vi "Recall Waveform to Reference Channel.vi"(7 "Waveform File":string, 8 "error in (no error)":errorcluster, 9 "Reference Channel (0: Reference 1)":i32(ring) items=["Reference 1", "Reference 2", "Reference 3", "Reference 4", "Edit Memory"], 10 "Source Waveform (0: Arbitrary Memory 1)":i32(ring) items=["Arbitrary Memory 1", "Arbitrary Memory 2", "Arbitrary Memory 3", "Arbitrary Memory 4", "Waveform File"], 11 "VISA resource name":refnum<visa-resource-name>) -> (0 "error out":errorcluster, 3 "VISA resource name out":refnum<visa-resource-name>)   [LabVIEW 2017, in "Scope.lvlib" / "Tektronix DPO MSO 2000 4000 Series.lvlib"]
doc: "Recalls a stored waveform to a reference memory location.\n\n<B>Notes:</B>\n(1) Only the first waveform in a .CSV file is recalled for multiple waveform .CSV files. \n\n(2) Recall of digital waveforms (D0 through D15) is not supported.\n\n(3) For MDO3000 series models, a saved ARB waveform cannot be recalled to a reference location. It can only be recalled to an EMEM location. However, an AFG waveform can be recalled into either a reference or EMEM location."
uses:
  Tektronix DPO MSO 2000 4000 Series.lvlib
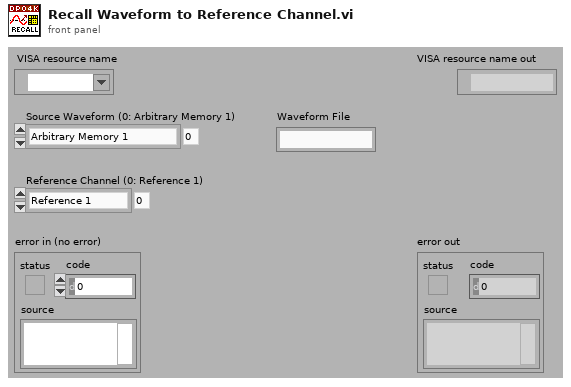
[diagram p1: front panel]
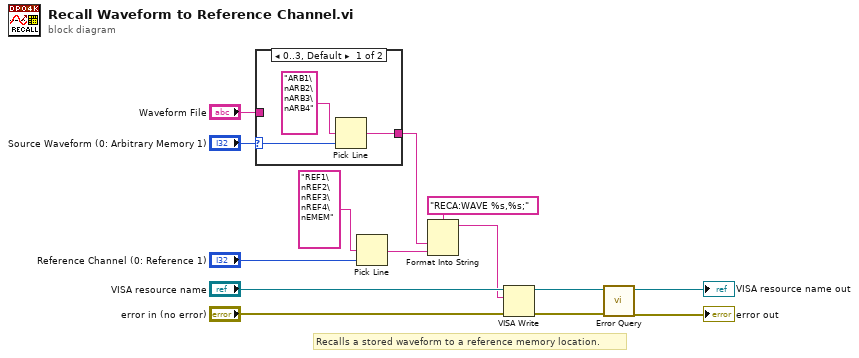
[diagram p0: block diagram]
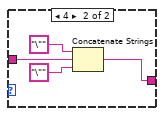
[diagram p2: hidden frame]
diagram:
  # "Recalls a stored waveform to a reference memory location."
  n1 = case shown="0..3, Default" "Source Waveform (0: Arbitrary Memory 1)" {
    selector: "Source Waveform (0: Arbitrary Memory 1)" -> [w16 _]
    tunnel: "Waveform File" -> [_ w21]
    tunnel: [w15 w18] -> w3
    frame 0..3, Default {
      n2 = Pick Line(multi-line string="ARB1\nARB2\nARB3\nARB4", line index=w16) -> (output string=w15:string)  [unwired: 1 in]
    }
    frame 4 {
      n3 = Concatenate Strings("\"" ("string"), w21, "\"" ("string")) -> (w18:string)
    }
  }
  n4 = Pick Line(multi-line string="REF1\nREF2\nREF3\nREF4\nEMEM", line index="Reference Channel (0: Reference 1)") -> (output string=w2:string)  [unwired: 1 in]
  n5 = Format Into String(format string="RECA:WAVE %s,%s;", w3, w2) -> (resulting string=w1:string)  [unwired: 2 in, 1 out]
  n6 = VISA Write(VISA resource name="VISA resource name", write buffer=w1, error in (no error)="error in (no error)") -> (VISA resource name out=w13:refnum<visa-resource-name>, error out=w12:errorcluster)  [unwired: 1 out]
  n7 = call "Error Query.vi"("error in (no error)"=w12, "VISA resource name"=w13) -> ("error out"=→"error out":errorcluster, "VISA resource name out"=→"VISA resource name out":refnum<visa-resource-name>)  [unwired: 6 in, 2 out]
